vi "GetSource.vi"(6 "error in":errorcluster, 9 "RightShiftRegister in":refnum<class "RightShiftRegister.lvclass">) -> (0 "error out":errorcluster, 3 "RightShiftRegister out":refnum<class "RightShiftRegister.lvclass">, 4 "name":string)   [LabVIEW 2014, in "RightShiftRegister.lvclass"]
uses:
  RightShiftRegister.lvclass
  Terminal/Terminal.lvclass
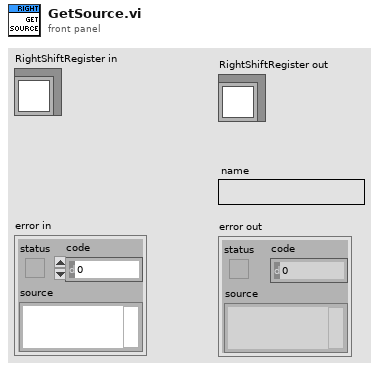
[diagram p1: front panel]
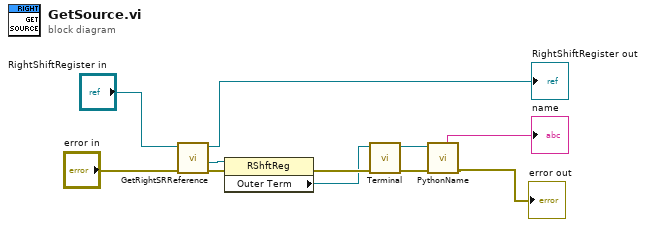
[diagram p0: block diagram]
diagram:
  n1 = call "GetRightSRReference.vi"("error in"="error in", "ShiftRegister in"="RightShiftRegister in") -> ("error out"=w7:errorcluster, "reference out"=w8:refnum<vi>, "ShiftRegister out"=→"RightShiftRegister out":refnum<class "RightShiftRegister.lvclass">)  [unwired: 7 in]
  n2 = property class="RShftReg"(reference=w8, error in=w7) -> (error out=w6:errorcluster, "Outer Term"=w5:refnum<vi>)  [unwired: 1 out]
  n3 = call "Terminal.vi"("error in"=w6, "refnum"=w5) -> ("error out"=w3:errorcluster, "terminal"=w4:refnum<class "Terminal.lvclass">)  [unwired: 8 in]
  n4 = call-dynamic "PythonName.vi"("error in"=w3, "Terminal in"=w4) -> ("error out"=→"error out":errorcluster, "name"=→"name":string)  [unwired: 6 in, 2 out]
